vi "Get Cell Value.vi"(7 "Sheet Name":string, 8 "error in":errorcluster, 10 "Cell Address":string, 11 "SpreadsheetDoc in":refnum<k24>) -> (0 "error out":errorcluster, 1 "Type":T1=enum."Boolean", 2 "Cell Value":T2 {"Timestamp" format="%<%x %.3X>T"}, 3 "SpreadsheetDoc out":refnum<k24>)   [LabVIEW 2019, in "Open Xml.lvlib"]
uses:
  Open Xml.lvlib
  D:/git/Open-Xml-LabVIEW/Source/DocumentFormat.OpenXml.dll
  DocumentFormat.OpenXml.dll
  Cell DataType.ctl
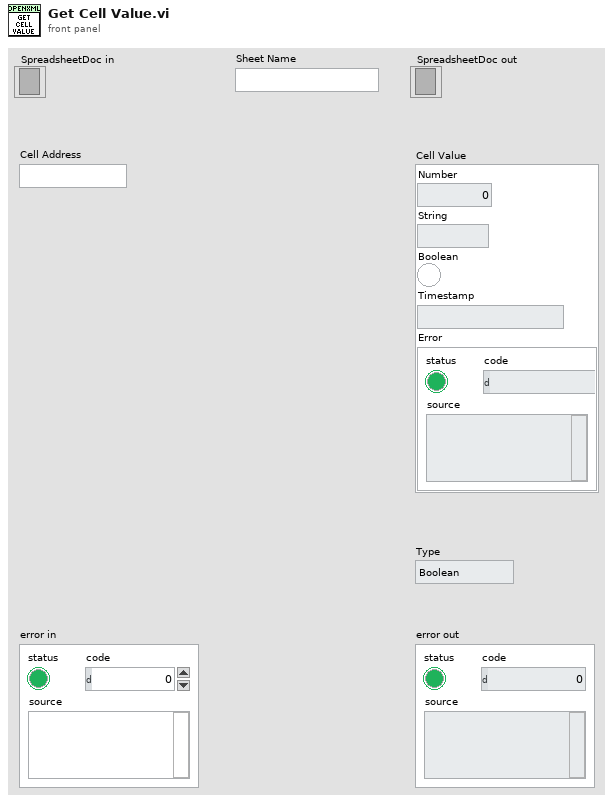
[diagram p1: front panel]
types:
  T1 = typedef "Open Xml.lvlib/Cell DataType.ctl" = enum16{"Void", "Boolean", "Number", "Error", "SharedString", "String", "InlineString", "Date"}
  T2 = cluster{"Number":dbl, "String":string, "Boolean":bool, "Timestamp":timestamp, "Error":errorcluster}
  T3 = cluster{"Number":dbl, "String":string, "Boolean":bool, "Time Stamp":timestamp, "Error":errorcluster}
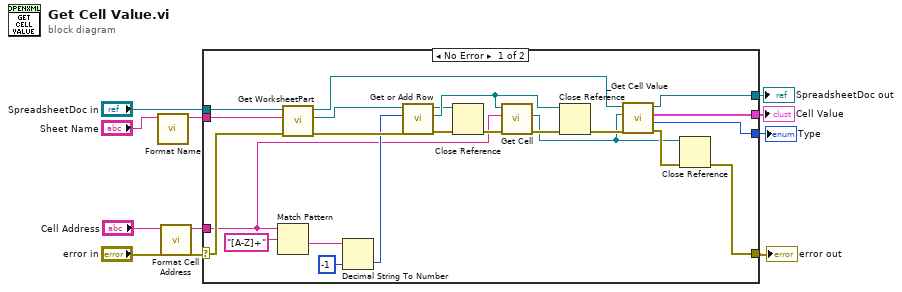
[diagram p0: block diagram]
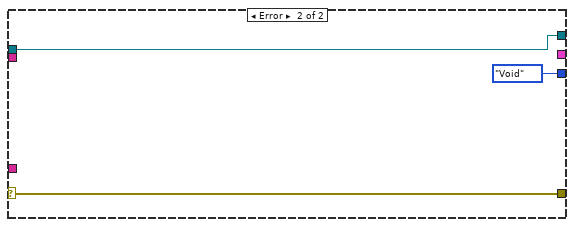
[diagram p2: hidden frame]
diagram:
  n1 = call "Format Name.vi"("Sheet Name"="Sheet Name") -> ("Formatted Sheet Name"=w2:string)  [unwired: 10 in]
  n2 = call "Format Cell Address.vi"("Cell Address"="Cell Address") -> ("Formatted Cell Address"=w5:string)  [unwired: 10 in]
  n3 = case shown="No Error" "error in" {
    selector: "error in" -> [w32 w36]
    tunnel: w2 -> [w33 _]
    tunnel: w5 -> [w11 _]
    tunnel: [w31 w36] -> w4
    tunnel: "SpreadsheetDoc in" -> [w30 w35]
    tunnel: [w29 w35] -> w8
    tunnel: [w28 Cell_DataType."Void" ("Type")] -> w6
    tunnel: [w27 _] -> w7
    frame No Error {
      n4 = Match Pattern(string=w11, regular expression="[A-Z]+") -> (after substring=w13:string)  [unwired: 1 in, 3 out]
      n5 = call "Get WorksheetPart.vi"("error in"=w32, "Sheet Name"=w33, "SpreadsheetDoc in"=w30) -> ("error out"=w26:errorcluster, "WorksheetPart"=w22:refnum<k24>, "SpreadsheetDoc out"=w18:refnum<k24>)  [unwired: 5 in, 1 out]
      n6 = Decimal String To Number(string=w13, default (0L)=i64 -1 ("default (0 I32)")) -> (number=w12:i64)  [unwired: 1 in, 1 out]
      n7 = call "Get or Add Row.vi"("error in"=w26, "Row Index"=w12, "Worksheetpart in"=w22) -> ("error out"=w23:errorcluster, "Row"=w21:refnum<k24>, "WorksheetPart out"=w16:refnum<k24>)  [unwired: 6 in]
      n8 = Close Reference(reference=w16, error in (no error)=w23) -> (error out=w24:errorcluster)
      n9 = call "Get Cell.vi"("error in"=w24, "Cell Address"=w11, "Row in"=w21) -> ("error out"=w25:errorcluster, "Cell"=w17:refnum<k24>)  [unwired: 6 in, 1 out]
      n10 = Close Reference(reference=w21, error in (no error)=w25) -> (error out=w20:errorcluster)
      n11 = call "_Get Cell Value.vi"("error in"=w20, "Cell"=w17, "SpreadsheetDoc in"=w18) -> ("error out"=w19:errorcluster, "Type"=w28:T1, "Cell Value"=w27:T3, "SpreadsheetDocument out"=w29:refnum<k24>)  [unwired: 5 in]
      n12 = Close Reference(reference=w17, error in (no error)=w19) -> (error out=w31:errorcluster)
    }
    frame Error {
    }
  }
  "SpreadsheetDoc out" <- w8
  "Cell Value" <- w7
  "Type" <- w6
  "error out" <- w4
